vi "LCP Set Fill Level.vi"(8 "error in (no error)":errorcluster caption="Fehler (Eingang, kein Fehler)", 9 "Flow":dbl, 10 "Level":dbl, 11 "Pump Handle":i64) -> (0 "error out":errorcluster caption="Fehler (Ausgang)")   [LabVIEW 2023, in "labbCAN_Pump_API.lvlib"]
doc: "LCP_Func long LCP_CALL LCP_SetFillLevel(dev_hdl hPump,\n double Level,\n double Flow);"
uses:
  labbCAN_Pump_API.lvlib
  labbCAN_Pump_API.dll
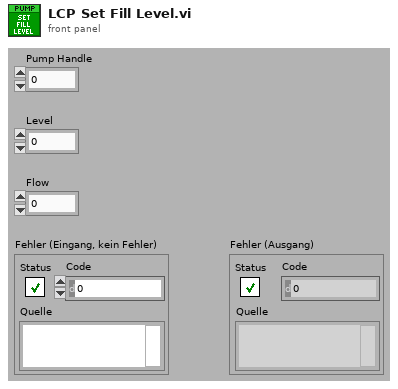
[diagram p1: front panel]
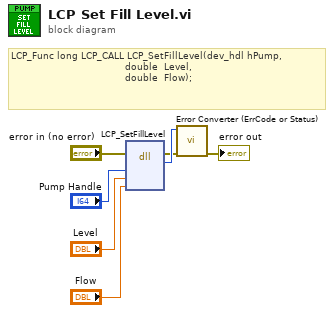
[diagram p0: block diagram]
diagram:
  # "LCP_Func long LCP_CALL LCP_SetFillLevel(dev_hdl hPump,\n\t                                     double  Level,\n\t                                     double  Flow);"
  n1 = dll-call lib="C:/GIT/AutomatedSetupAcousticEnergyDensity/CETONI_SDK/labbCAN_Pump_API.*" fn="LCP_SetFillLevel"(error in="error in (no error)", "hPump"="Pump Handle", "Level"="Level", "Flow"="Flow") -> (error out=w2:errorcluster, "Rückgabetyp"=w3:i32)  [unwired: 5 in, 1 out]
  n2 = call "Error Converter (ErrCode or Status).vi"("error in (no error)"=w2, "error code"=w3) -> ("error out"=→"error out":errorcluster)  [unwired: 9 in]
